vi "GroupUI.vi"() -> ()   [LabVIEW 2013, in "Group.lvclass"]
uses:
  Group.lvclass
  CEF_TreeControl/Node/NodeRef.ctl
  CEF_TreeControl/Node/NISE_CEF_Node.lvclass
  <vilib>/NI/AMC/Message Queue.ctl
  <vilib>/NI/AMC/Message.ctl
  <vilib>/NI/Tools/Keyed Array/KeyedArray.ctl
  CEF_TreeControl/Node/UserEventRef.ctl
  CEF_TreeControl/Controls/EventCluster.ctl
  Group.lvclass/Group.ctl
  Read GroupName.vi
  Write GroupName.vi
  <vilib>/NI/AMC/Create Single Message.vi
  <vilib>/NI/AMC/Update Message Routing Info.vi
  <vilib>/NI/AMC/Send Message.vi
  <vilib>/NI/AMC/AMC.lvlib
  <vilib>/NI/Tools/Keyed Array/Tools_KeyedArray.lvlib
  CEF_TreeControl/NISE_CEF_TreeControl.lvlib
panel:
  in  "user event":T1
  in  "main queue":T2
  in  "Group Name":string
  in  "node ref":T3
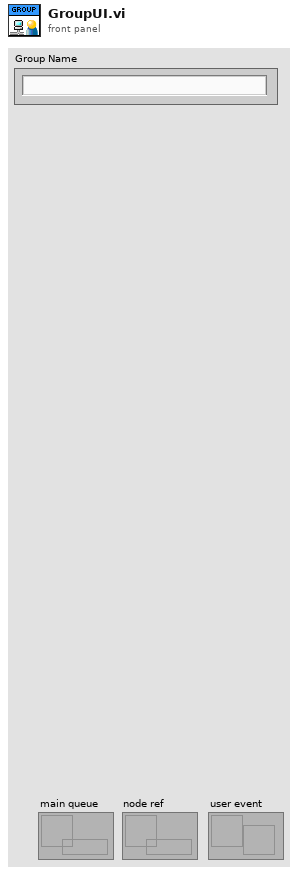
[diagram p1: front panel]
types:
  T1 = typedef "NISE_CEF_Node.lvclass/UserEventRef.ctl" = refnum<user-event>
  T2 = typedef "AMC.lvlib/Message Queue.ctl" = refnum<queue>
  T3 = typedef "NISE_CEF_Node.lvclass/NodeRef.ctl" = refnum<data-value>
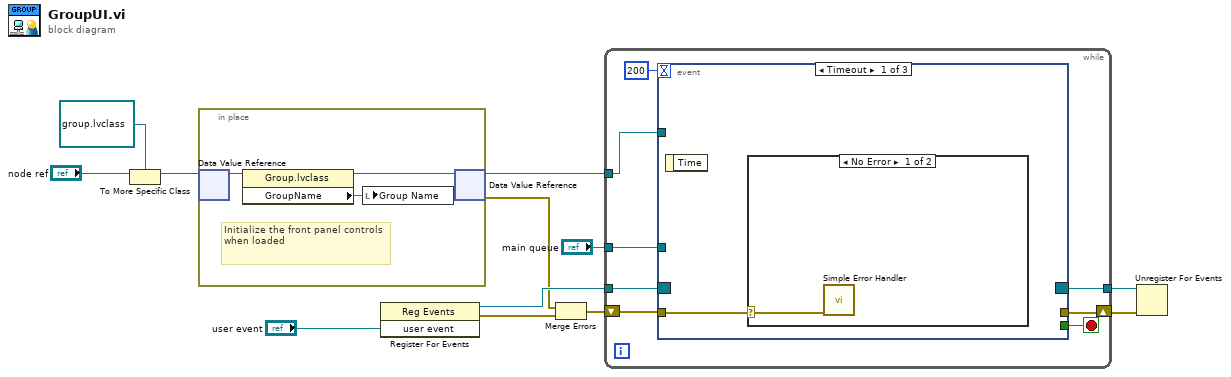
[diagram p0: block diagram]
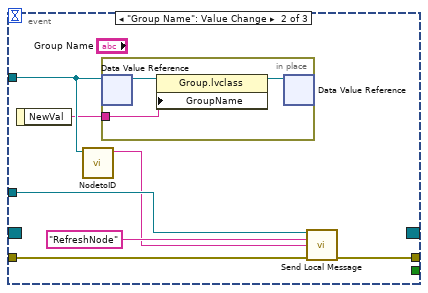
[diagram p3: hidden frame]
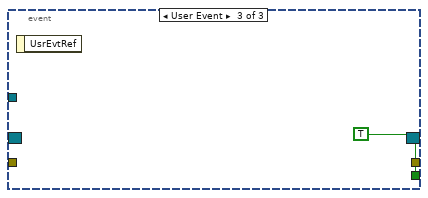
[diagram p4: hidden frame]
diagram:
  n1 = To More Specific Class(target class=refnum<data-value> refnum ("data value reference"), reference="node ref") -> (specific class reference=w5:refnum<data-value>)  [unwired: 1 in, 1 out]
  n2 = in-place {
    # "Initialize the front panel controls when loaded"
    n3 = in-place-dvr #1(w5) -> (w15:refnum<class "Group.lvclass">)  [unwired: 1 out]
    n4 = property class="Group.lvclass"(reference=w15) -> (reference out=w14:refnum<class "Group.lvclass">, "GroupName"=w13:string)  [unwired: 1 in, 1 out]
    n5 = local write "Group Name"(w13) -> ()
    n6 = in-place-dvr #1(w14) -> (w12:refnum<data-value>, w2:errorcluster)
  }
  n7 = register-events("user event") -> (reference out=w9:refnum<event-registration>, error out=w3:errorcluster)  [unwired: 2 in]
  n8 = Merge Errors(w2, w3) -> (w1:errorcluster)
  n9 = while {
    tunnel: w12 -> [w23]
    tunnel: "main queue" -> [w22]
    tunnel: w9 -> [w20]
    tunnel: [w19] -> w8
    shift-right: [w17] -> w7
    shift-left: w1 -> [w16]
    stop <- w18 stop-if-true
    n10 = event shown="[0] Timeout" {
      selector: w20 -> [_ _ _]
      dyn-events: [_ _ _] -> w19
      timeout: 200 -> [_ _ _]
      tunnel: w23 -> [_ w30 _]
      tunnel: w22 -> [_ w31 _]
      tunnel: [_ _ TRUE] -> w18
      tunnel: [_ w28 _] -> w17
      tunnel: w16 -> [w24 w27 _]
      event Timeout {
        n11 = event-data() -> ()  [unwired: 1 in, 1 out]
        n12 = case shown="No Error" w24 {
          selector: w24 -> [w25 _]
          frame No Error {
            n13 = call <vilib>:"Simple Error Handler.vi"("error in (no error)"=w25) -> ()  [unwired: 4 in, 5 out]
          }
          frame Error {
          }
        }
      }
      event "Group Name": Value Change {
        n14 = event-data() -> ("NewVal"=w26:string)  [unwired: 1 in]
        n15 = call "NodetoID.vi"("node ref"=w30) -> ("ID"=w29:string)  [unwired: 9 in, 1 out]
        n16 = in-place {
          in-place-border: w26 -> [w33]
          n17 = in-place-dvr #2(w30) -> (w35:refnum<class "Group.lvclass">)  [unwired: 1 out]
          n18 = property class="Group.lvclass"(reference=w35, "GroupName"=w33) -> (reference out=w34:refnum<class "Group.lvclass">)  [unwired: 1 in, 1 out]
          n19 = in-place-dvr #2(w34) -> ()  [unwired: 2 out]
        }
        n20 = call <vilib>:"Send Local Message.vi"("message queue in"=w31, "message name"="RefreshNode" ("Message Name"), "message value"=w29, "error in"=w27) -> ("error out"=w28:errorcluster)  [unwired: 9 in, 2 out]
      }
      event User Event {
        n21 = event-data() -> ()  [unwired: 1 in, 1 out]
      }
    }
  }
  n22 = Unregister For Events(event registration refnum=w8, error in=w7) -> ()  [unwired: 1 out]
